vi "Hide FGV.vi"(6 "Command":T1, 8 "Hide":bool) -> (0 "Hide?":bool)   [LabVIEW 2015]
uses:
  TypeDefs Dani/Open Audio FGV Enum Dani.ctl
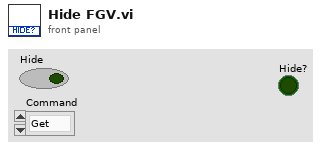
[diagram p1: front panel]
types:
  T1 = typedef "Open Audio FGV Enum Dani.ctl" = enum16{"Get", "Set"}
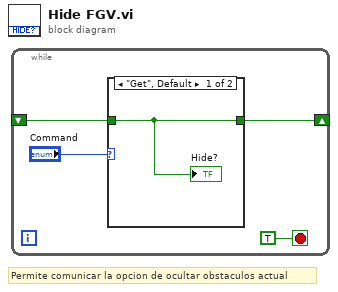
[diagram p0: block diagram]
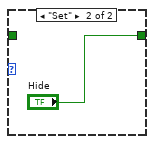
[diagram p2: hidden frame]
diagram:
  # "Permite comunicar la opcion de ocultar obstaculos actual"
  n1 = while {
    shift-right: [w2] -> _
    shift-left: _ -> [w1]
    stop <- TRUE stop-if-true
    n2 = case shown="\"Get\", Default" "Command" {
      tunnel: [w5 "Hide"] -> w2
      tunnel: w1 -> [w5 _]
      frame "Get", Default {
        "Hide?" <- w5
      }
      frame "Set" {
      }
    }
  }
